vi "Configuration List Operation.vi"(8 "error in (no error)":errorcluster, 9 "Name (\"\")":string, 10 "List Operation (0: Delete)":i32(ring) items=["Create", "Delete", "Recall", "Store"], 11 "VISA resource name":refnum<visa-resource-name>) -> (0 "error out":errorcluster, 3 "VISA resource name out":refnum<visa-resource-name>)   [LabVIEW 2023, in "Keithley DMM6500 DAQ6500 Series.lvlib"]
doc: "Creates, deletes, recalls or stores a configuration list."
uses:
  <instrlib>/Keithley DMM6500 DAQ6500 Series/Keithley DMM6500 DAQ6500 Series.lvlib
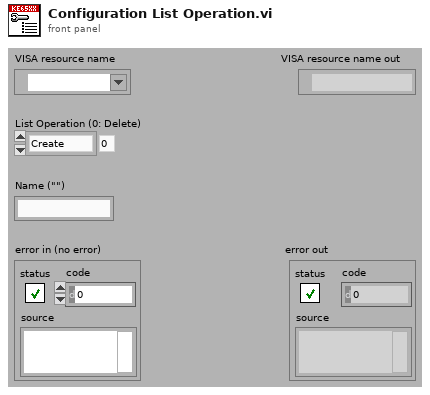
[diagram p1: front panel]
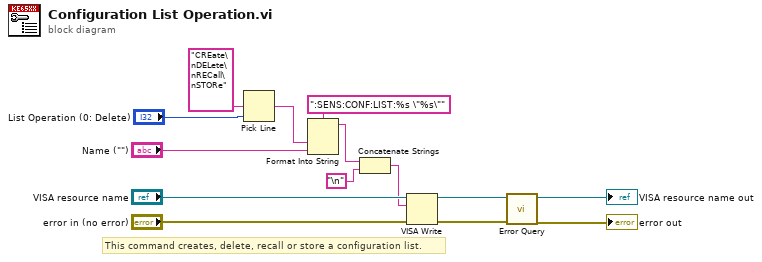
[diagram p0: block diagram]
diagram:
  # "This command creates, delete, recall or store a configuration list."
  n1 = Pick Line(multi-line string="CREate\nDELete\nRECall\nSTORe", line index="List Operation (0: Delete)") -> (output string=w3:string)  [unwired: 1 in]
  n2 = Format Into String(format string=":SENS:CONF:LIST:%s \"%s\"", w3, "Name (\"\")") -> (resulting string=w5:string)  [unwired: 2 in, 1 out]
  n3 = Concatenate Strings(w5, "\n") -> (w6:string)
  n4 = VISA Write(VISA resource name="VISA resource name", write buffer=w6, error in (no error)="error in (no error)") -> (VISA resource name out=w10:refnum<visa-resource-name>, error out=w9:errorcluster)  [unwired: 1 out]
  n5 = call <instrlib>:"Error Query.vi"("error in (no error)"=w9, "VISA resource name"=w10) -> ("error out"=→"error out":errorcluster, "VISA resource name out"=→"VISA resource name out":refnum<visa-resource-name>)  [unwired: 6 in, 2 out]
